vi "Add Source Path if Error.vi"(6 "Upstream Error":errorcluster, 7 "Source Path or URL":string, 8 "error in (no error)":errorcluster) -> (0 "error out":errorcluster)   [LabVIEW 2020, in "JKI JSON Serialization.lvlib"]
doc: "If error occurred deserializing or writing JSON to disk, AND no Upstream Error exists, Soure Path or URL will be inserted into the error description."
uses:
  JKI JSON Serialization.lvlib
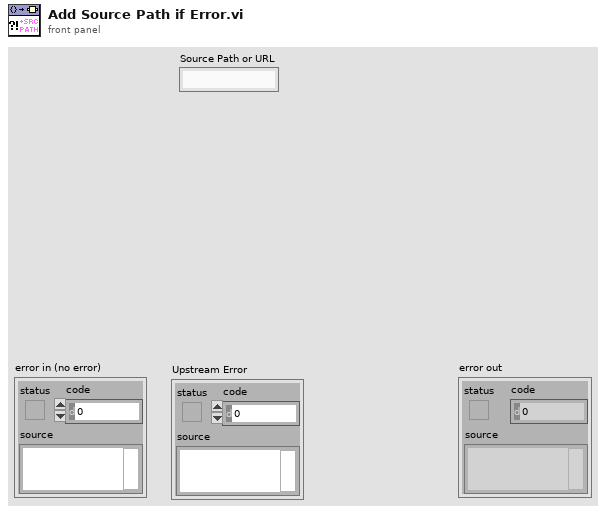
[diagram p1: front panel]
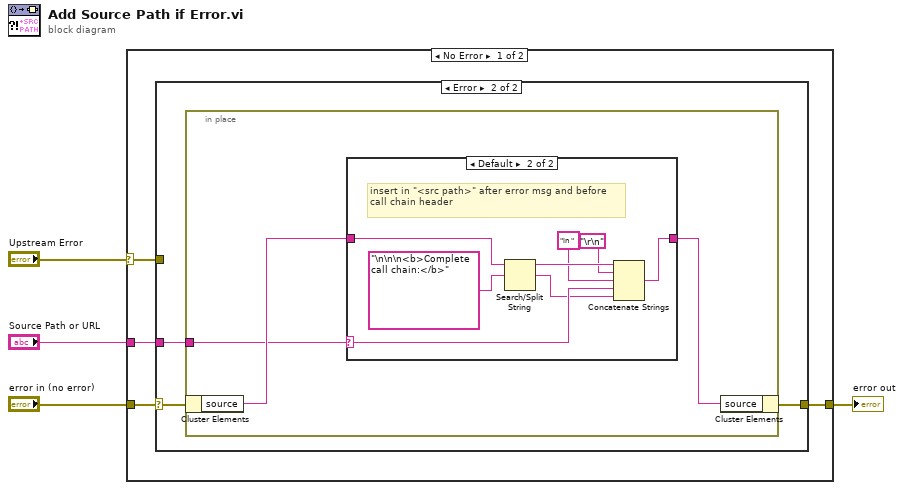
[diagram p0: block diagram]
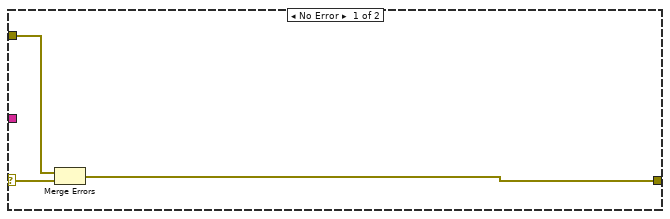
[diagram p2: hidden frame]
diagram:
  n1 = case shown="No Error" "Upstream Error" {
    selector: "Upstream Error" -> [w5 w27]
    tunnel: "error in (no error)" -> [w8 _]
    tunnel: [w7 w27] -> w3
    tunnel: "Source Path or URL" -> [w6 _]
    frame No Error {
      n2 = case shown="Error" w8 {
        selector: w8 -> [w11 w14]
        tunnel: [w10 w13] -> w7
        tunnel: w6 -> [_ w12]
        tunnel: w5 -> [w9 _]
        frame No Error {
          n3 = Merge Errors(w9, w11) -> (w10:errorcluster)
        }
        frame Error {
          n4 = in-place {
            in-place-border: w12 -> [w15]
            n5 = in-place-cluster #1(w14) -> ("source"=w17:string)
            n6 = case shown="Default" w15 {
              selector: w15 -> [_ w22]
              tunnel: w17 -> [w18 w25]
              tunnel: [w18 w20] -> w16
              frame "" {
              }
              frame Default {
                # "insert in \"<src path>\" after error msg and before call chain header"
                n7 = Search/Split String(string=w25, search string/char (-)="\n\n\n<b>Complete call chain:</b>") -> (substring before match=w24:string, match + rest of string=w21:string)  [unwired: 1 in, 1 out]
                n8 = Concatenate Strings(w24, "\r\n", "in " ("string"), w22, w21) -> (w20:string)
              }
            }
            n9 = in-place-cluster #1("source"=w16) -> (w13:errorcluster)
          }
        }
      }
    }
    frame Error {
    }
  }
  "error out" <- w3
